vi "weighPlatformsV1.vi"(11 "DAQmx Physical Channel":tag="Dev2/ai0:31") -> (3 "load cell\nsignal":dbl[](array[numeric]))   [LabVIEW 2017]
doc: "Measures the voltage output by the load cell across all the selected channels.\nMultiple samples are taken, filtered and then averaged. \nDuration of measurement is hard-wired."
uses:
  <vilib>/Analysis/3filter.llb/Filter Passband Type.ctl
  <vilib>/DAQmx/read.llb/DAQmx Read (Analog 2D DBL NChan NSamp).vi
  <vilib>/Analysis/baseanly.llb/Mean (DBL).vi
  <vilib>/DAQmx/create/channels.llb/DAQmx Create Channel (AI-Voltage-Basic).vi
  <vilib>/DAQmx/configure/timing.llb/DAQmx Timing (Sample Clock).vi
  <vilib>/DAQmx/miscellaneous.llb/DAQmx Fill In Error Info.vi
  <vilib>/Analysis/3filter.llb/Butterworth Filter (DBL).vi
  <vilib>/Analysis/NI_AALBase.lvlib
panel:
  in  "sample mode":i32(ring)=10178 items=["Finite Samples"=10178, "Continuous Samples"=10123, "Hardware Timed Single Point"=12522]
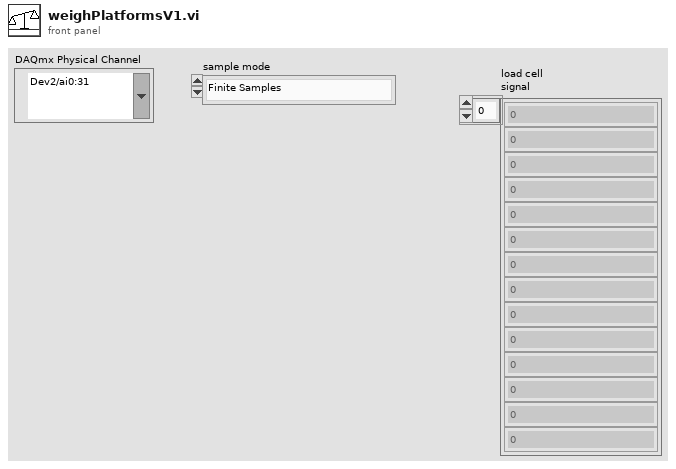
[diagram p1: front panel]
types:
  T1 = typedef "NI_AALBase.lvlib/Filter Passband Type.ctl" = enum32{"Lowpass", "Highpass", "Bandpass", "Bandstop"}
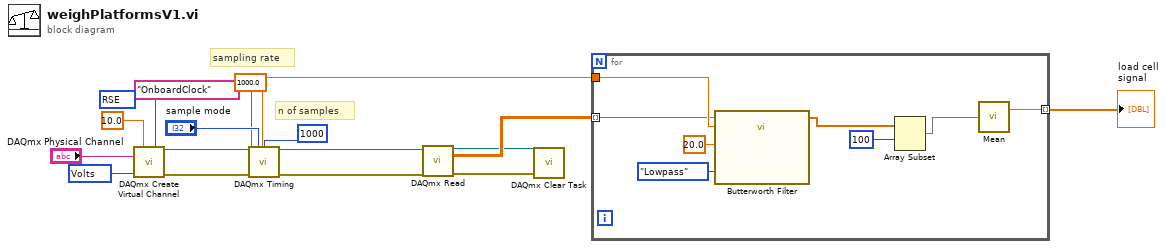
[diagram p0: block diagram]
diagram:
  w4 = 10348 items=["Volts"=10348, "From Custom Scale"=10065] ("units")
  w5 = 10083 items=["Default"=-1, "RSE"=10083, "NRSE"=10078, "Differential"=10106, "Pseudodifferential"=12529] ("input terminal configuration")
  w9 = 1000.0 ("rate")
  # "n of samples"
  # "sampling rate"
  n1 = call-poly <vilib>:"DAQmx Create Virtual Channel.vi"("maximum value"=10.0, "input terminal configuration"=w5, "physical channels"="DAQmx Physical Channel", "units"=w4) -> ("task out"=w16:refnum<k21>, "error out"=w13:errorcluster)  [unwired: 10 in]
  n2 = call-poly <vilib>:"DAQmx Timing.vi"("task/channels in"=w16, "sample mode"="sample mode", "samples per channel"=1000, "rate"=w9, "source"=tag "OnboardClock", "error in"=w13) -> ("task out"=w14:refnum<k21>, "error out"=w12:errorcluster)  [unwired: 8 in]
  n3 = call-poly <vilib>:"DAQmx Read.vi"("task/channels in"=w14, "error in"=w12) -> ("task out"=w7:refnum<k21>, "data"=w11:dbl[][], "error out"=w6:errorcluster)  [unwired: 11 in]
  n4 = call <vilib>:"DAQmx Clear Task.vi"("task in"=w7, "error in"=w6) -> ()  [unwired: 13 in, 1 out]
  n5 = for {
    tunnel: w11 -> [w23] mode=indexing
    tunnel: w9 -> [w24]
    tunnel: [w22] -> w1 mode=indexing
    n6 = call-poly <vilib>:"Butterworth Filter.vi"("filter type"=Filter_Passband_Type."Lowpass", "low cutoff freq: fl"=20.0, "sampling freq: fs"=w24, "X"=w23) -> ("Filtered X"=w18:dbl[])  [unwired: 4 in, 1 out]
    n7 = Array Subset(array=w18, index=100) -> (w17:dbl[])  [unwired: 1 in]
    n8 = call-poly <vilib>:"Mean.vi"("X"=w17) -> ("mean"=w22:dbl)  [unwired: 1 out]
  }
  "load cell\nsignal" <- w1
